vi "KioskDemoHoriz.vi"() -> ()   [LabVIEW 2023]
doc: "DESCRIPTION\nGeneral Application \n\nVERSION\nD1:00\nFirst Release To customer\nDD/MM/YYYY\n\nTemplate D2:01\nMade lighter and simpler\n14-04-2020"
uses:
  SubVIs/Controls/SetupModeState.ctl
  <vilib>/event_ctls.llb/eventsource.ctl
  <vilib>/Utility/miscctls.llb/LVBoundsTypeDef.ctl
  SubVIs/Controls/DisplayQCommand.ctl
  SubVIs/Controls/QueueCommand.ctl
  SubVIs/Controls/DisplayMessage.ctl
  SubVIs/Controls/Transition.ctl
  SubVIs/utilities/Error/ErrorCommand.ctl
  SubVIs/Controls/Tab.ctl
  SubVIs/Controls/StateMessage.ctl
  SubVIs/Error/ErrorMessage.ctl
  SubVIs/utilities/Config/System Config Data Manager Parameter.ctl
  SubVIs/utilities/Config/ConfigCommand.ctl
  SubVIs/Buttons/ButtonCommands.ctl
  SubVIs/Buttons/MenuType.ctl
panel:
  in  "Position:Top":i32
  in  "exit":bool
  in  "Container Bounds":T1
  out "Application Directory":path
  in  "ButtonsMenu":enum32{"Page 1"}(tab)
  out "SubmenuVisible":bool
  out "State":T2=enum."Initialising"
  out "UI Output":string
  out "Menu Output":string
  in  "Tab Control 2":enum32{"Page 1", "Page 4", "Page 2", "Page 3"}(tab)
  in  "Stop":bool
  in  "Source":T3 items=["LabVIEW UI"=0, "ActiveX"=1, "User Event"=25]
  in  "Start":bool
  out "ErrorHandlingLoop":i32
  out "StateMachineLoop":i32
  out "UILoop":i32
  out "EventLoop":i32
  in  "Main Screen Tabs":enum32{"Main Screen"}(tab)
  out "Tab Control":T4(tab)
  in  "Error Loop":enum16{"Event Loop", "UI Q Loop", "State Loop"}(ring)
  in  "Generate Error":bool
  out "EngMode?":bool
  in  "Enter Password":string
  out "ConfigdB path":path
  in  "Home Button":bool
  in  "ErrorLog":bool
  in  "Clear Alarm":bool
  in  "ErrorLog":i32(listbox)
  out "Error":string
  out "ErrorIndicator":bool
  in  "ViewError":bool
  out "Version":string
  out "Time":string
  out "Status":string
  # "GenAppMain"
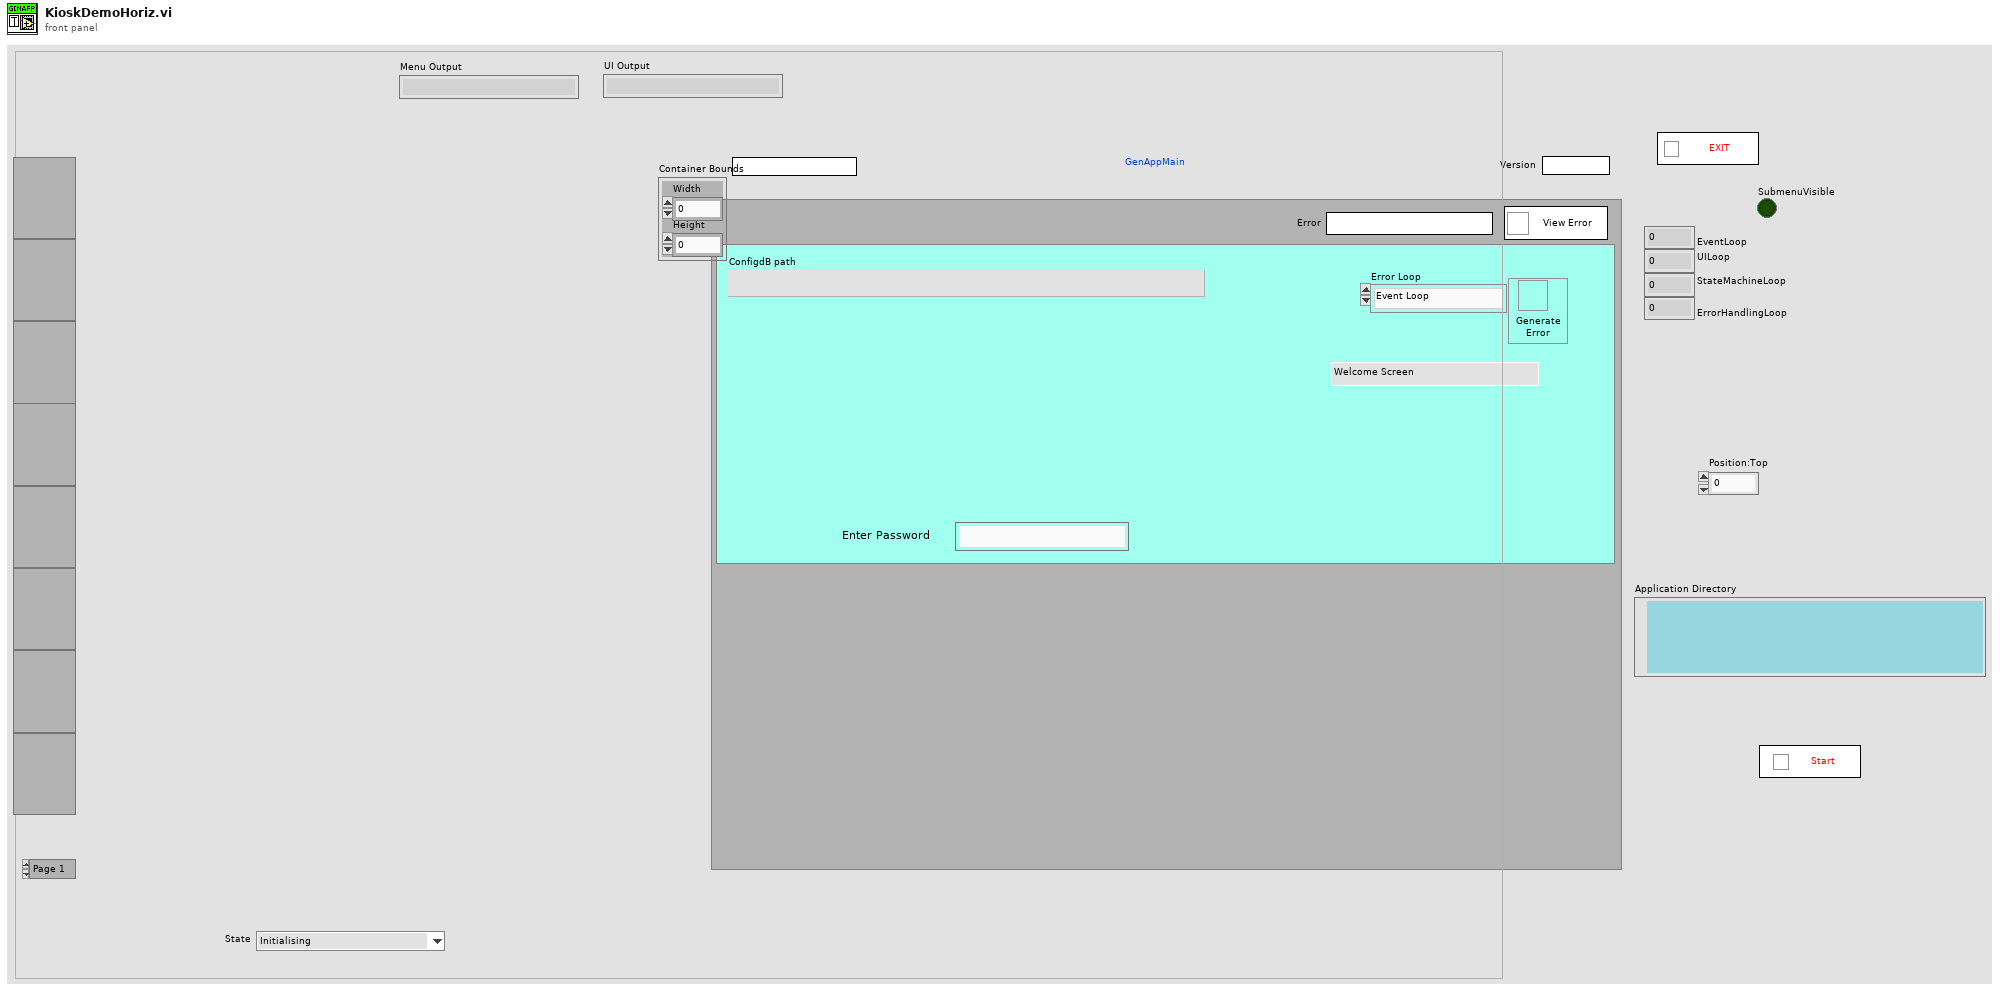
[diagram p1: front panel]
types:
  T1 = typedef "LVBoundsTypeDef.ctl" = cluster{"Width":u32, "Height":u32}
  T2 = typedef "SetupModeState.ctl" = enum16{"No State - Error", "Initialising", "Idling", "Running", "Sorting Menu", "Resetting Menu", "Sorting Submenu", "Loading UI", "Erroring", "Exiting"}
  T3 = typedef "eventsource.ctl" = u32
  T4 = enum32{"Welcome Screen", "Eng Set Up", "Oppo Run Screen", "Eng Run Screen", "Test Report Screen", "Error"}
  T5 = typedef "DisplayQCommand.ctl" = enum16{"No Command - Error", "Initialise", "Get Q Reference", "Add Item to Bottom", "Add Item to Top", "Flush Q", "Dequeue", "Peek Next Element", "Close"}
  T6 = typedef "QueueCommand.ctl" = enum16{"No Command - Error", "Initialise", "Add to Bottom", "Add To Top", "Get Ref", "Close"}
  T7 = typedef "ErrorCommand.ctl" = enum16{"No Command - Error", "Set to Dev Mode", "Set To Released Mode", "Set Error", "Log Error", "Throw Error", "Log & Throw Error", "Set Error Timed"}
  T8 = enum32{"invalid app kind", "Development System", "Run Time System", "Student Edition", "Embedded LabVIEW", "Evaluation", "Custom"}
  T9 = typedef "DisplayMessage.ctl" = enum16{"No Message - Ignore", "Display Message", "Set Tab", "Set Status", "Add Error Message", "Clear Error History", "Generate Error", "Set Idling Display", "Set Running Display", "Set Subpanel Output", "Stop"}
  T10 = typedef "ErrorMessage.ctl" = enum16{"No Message - Ignore", "Display Message", "Stop"}
  T11 = typedef "StateMessage.ctl" = cluster{"Transition":T12, "variant":variant}
  T12 = typedef "Transition.ctl" = enum16{"No Transition - Error", "Initialise", "Login", "Authenticate", "Log on Fail", "Login Success", "Logout", "Generate Error", "Start", "Stop", "Menu Button Pressed", "UI Button Pressed", "Exit"}
  T13 = typedef "ConfigCommand.ctl" = enum16{"No Command - Error", "Initialise Config SQLite", "Save Config", "Get Key", "Set Key", "Update Key", "Get Latest Config Data", "Get Config Data for Version", "Get Default Config Data"}
  T14 = typedef "System Config Data Manager Parameter.ctl" = enum16{"Eng Password", "DSN Connection", "User Password", "RunStatus", "InitialDataPath", "helpFilePath", "ErrorFilepath", "DatalogPath", "Hello"}
  T15 = typedef "Tab.ctl" = enum32{"Welcome Screen", "Eng Set Up", "Oppo Run Screen", "Eng Run Screen", "Test Report Screen", "Error"}
  T16 = typedef "lveventtype.ctl" = enum32{"Null", "Timeout", "Annotation Menu Selection", "Annotation Menu Selection?", "App Instance Close", "App Instance Close?", "Autoscale Range Change", "Bookmark Info Change", "Cell Edit", "Cell Edit?", "Cursor Grab", "Cursor Grab?", "Cursor Menu Selection", "Cursor Menu Selection?", "Cursor Move", "Cursor Release", "Data Change", "Direction Change", "Display State Change", "Drag Ended", "Drag Enter", "Drag Leave", "Drag Over", "Drag Source Update", "Drag Starting", "Drag Starting?", "Drop", "Exec State Change", "Key Down", "Key Down?", "Key Repeat", "Key Repeat?", "Key Up", "Listbox Double Click", "Menu Activation?", "Menu Selection (App)", "Menu Selection? (App)", "Menu Selection (User)", "Mouse Down", "Mouse Down?", "Mouse Enter", "Mouse Leave", "Mouse Move", "Mouse Up", "Mouse Wheel", "NI Security User Change (App)", "Pane Size", "Panel Close", "Panel Close?", "Panel Resize", "Plot Attribute Change", "Scale Range Change", "Shortcut Menu Activation?", "Shortcut Menu Selection (App)", "Shortcut Menu Selection? (App)", "Shortcut Menu Selection (User)", "Tree Double Click", "Tree Drag", "Tree Drag?", "Tree Drop", "Tree Drop?", "Tree Item Close", "Tree Item Close?", "Tree Item Open", "Tree Item Open?", "User Event", "Value Change"}
  T17 = typedef "MenuType.ctl" = enum16{"Main", "Simulation", "ME", "SF", "User Utilities", "Dev Tools"}
  T18 = typedef "ButtonCommands.ctl" = enum16{"No Command - Error", "Load Buttons", "Remove Buttons"}
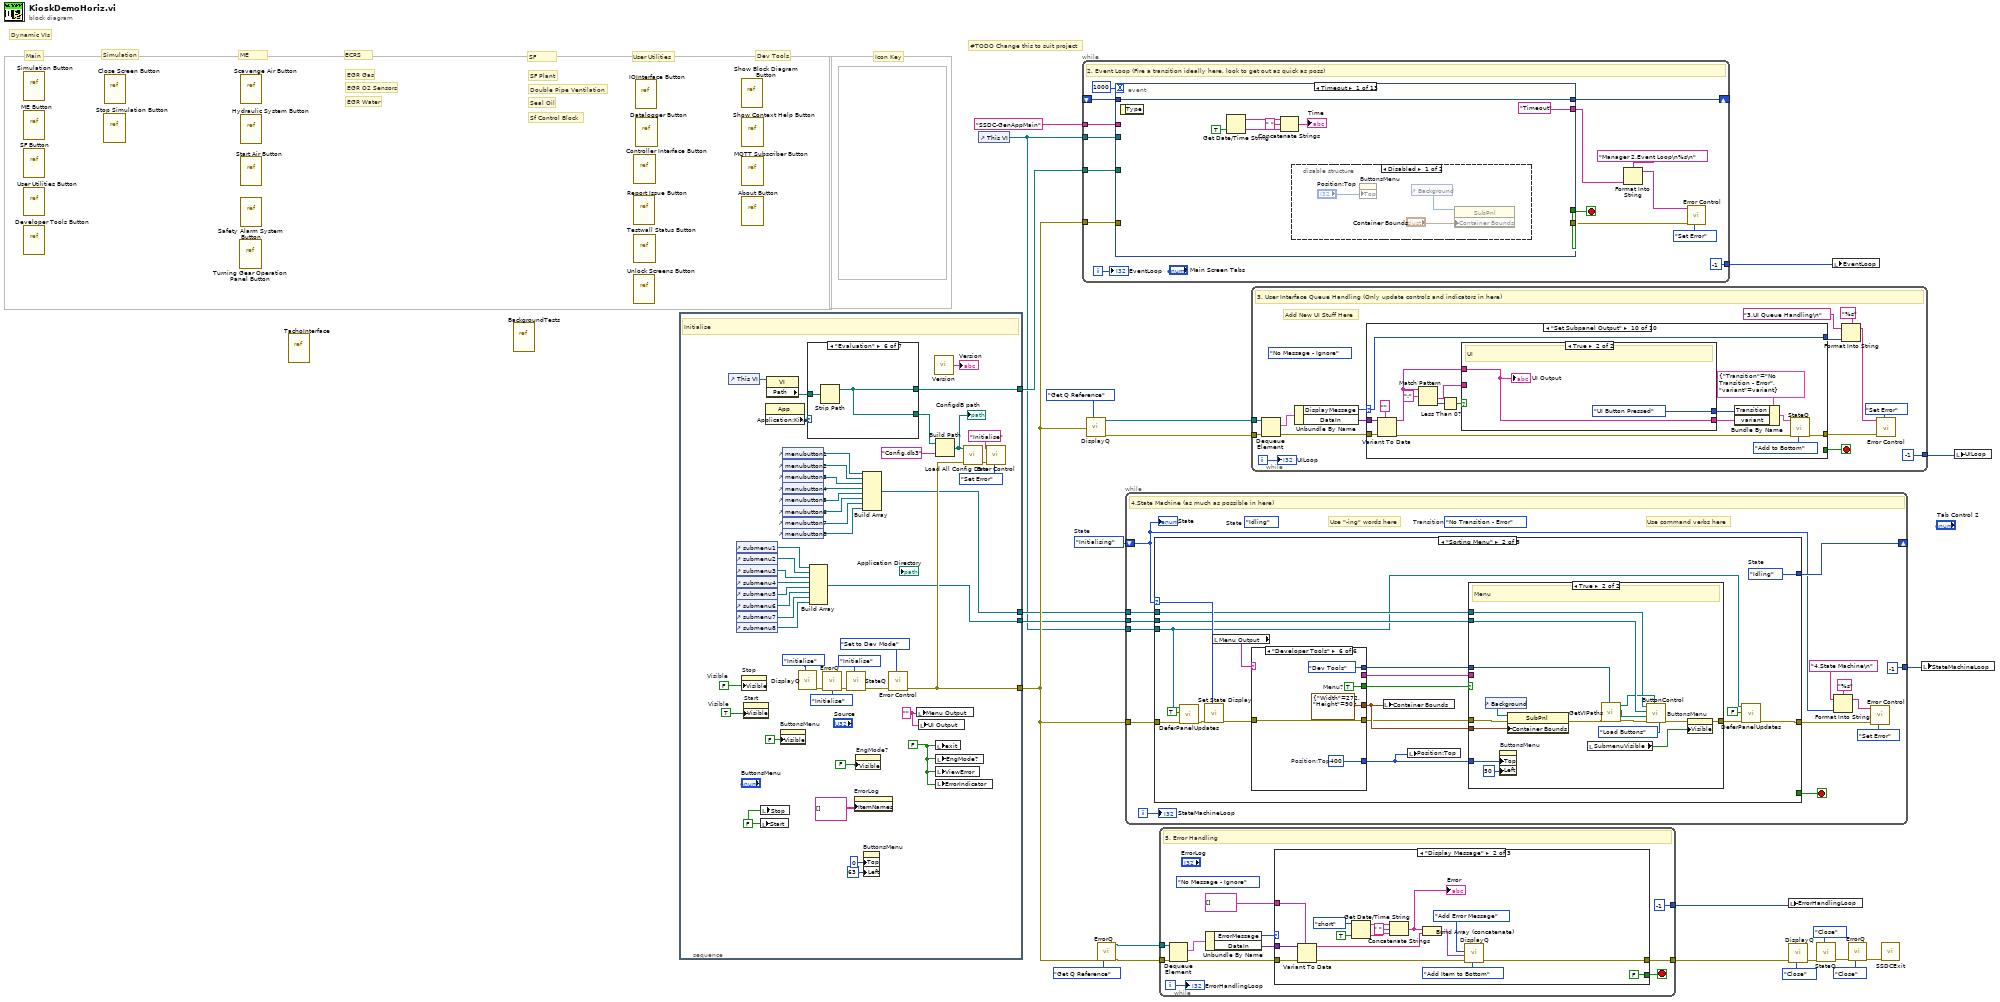
[diagram p0: block diagram]
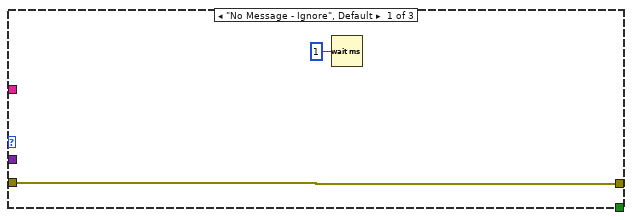
[diagram p2: hidden frame]
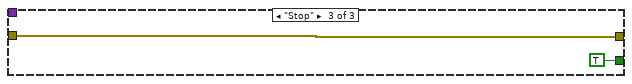
[diagram p3: hidden frame]
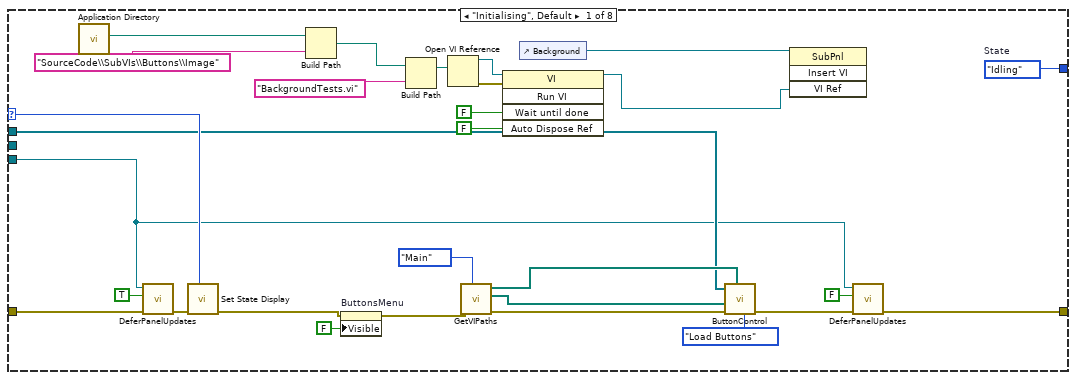
[diagram p4: hidden frame]
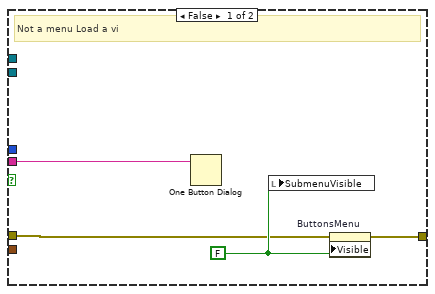
[diagram p5: hidden frame]
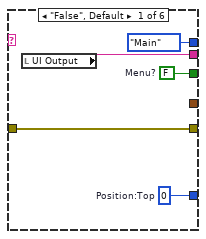
[diagram p6: hidden frame]
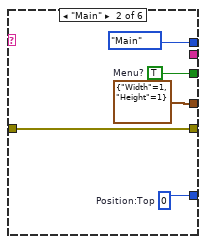
[diagram p7: hidden frame]
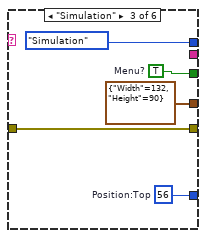
[diagram p8: hidden frame]
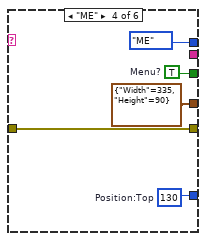
[diagram p9: hidden frame]
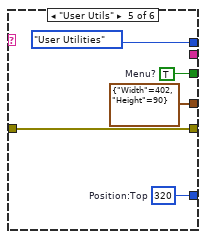
[diagram p10: hidden frame]
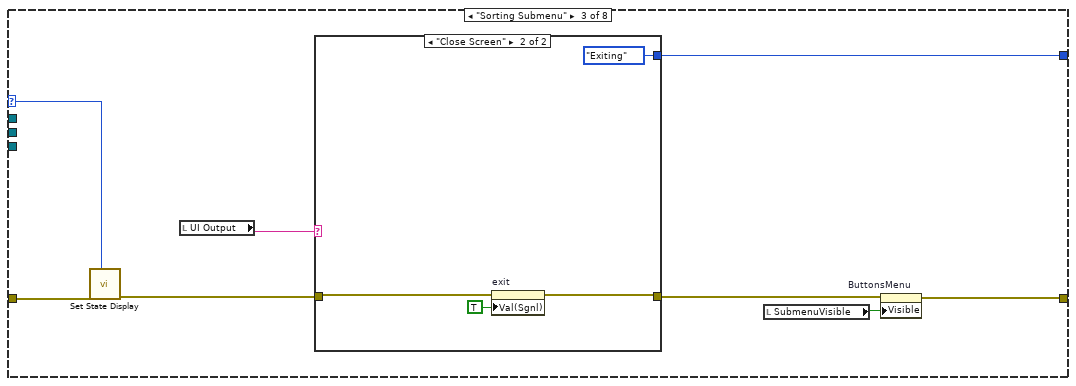
[diagram p11: hidden frame]
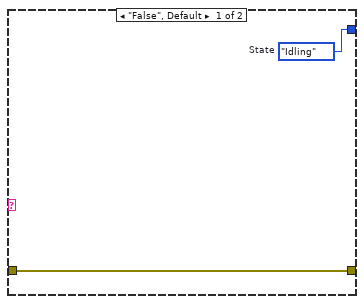
[diagram p12: hidden frame]
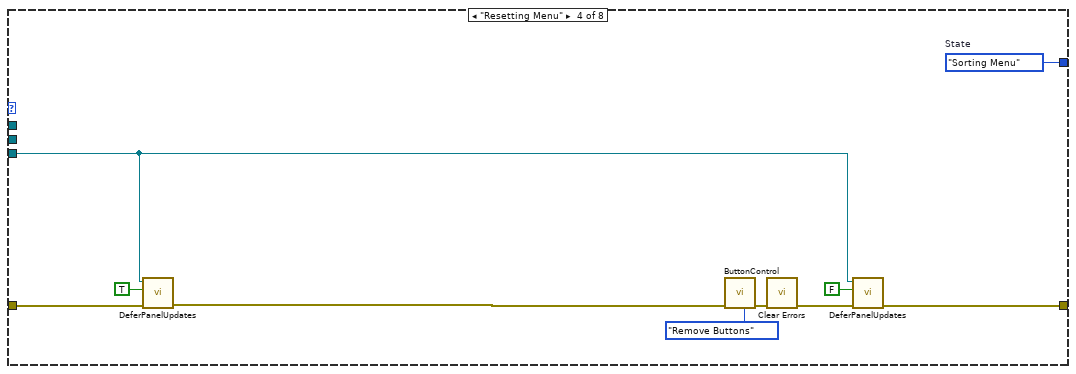
[diagram p13: hidden frame]
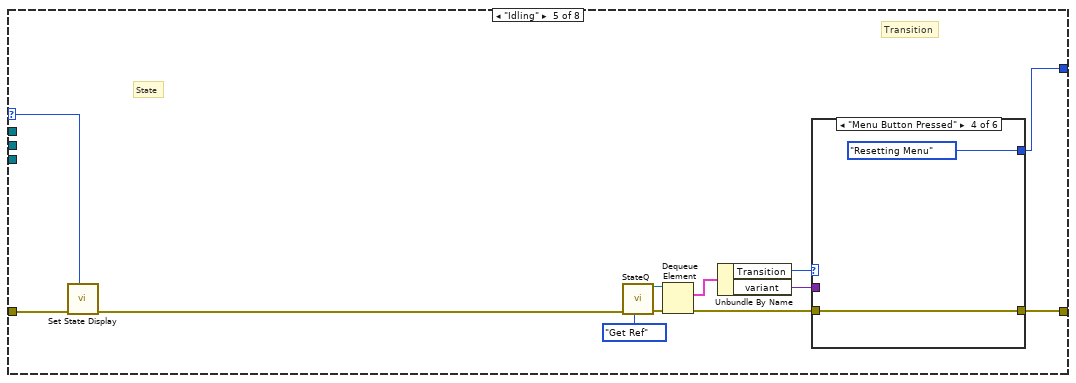
[diagram p14: hidden frame]
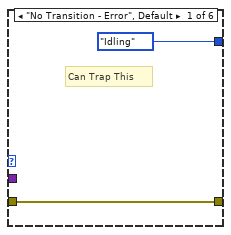
[diagram p15: hidden frame]
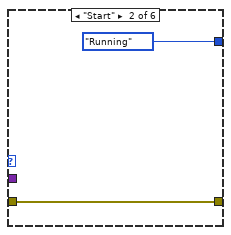
[diagram p16: hidden frame]
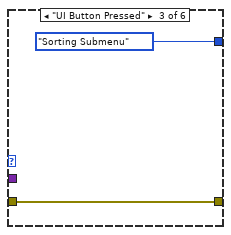
[diagram p17: hidden frame]
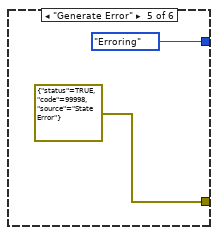
[diagram p18: hidden frame]
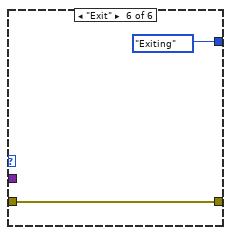
[diagram p19: hidden frame]
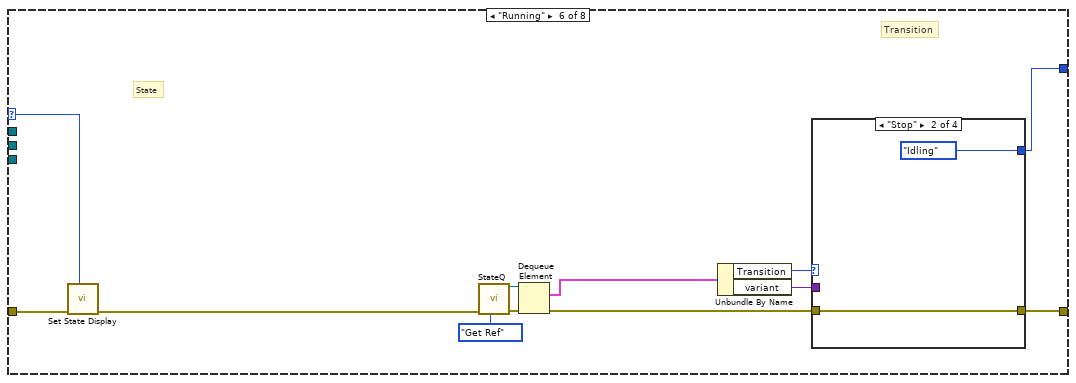
[diagram p20: hidden frame]
diagram:
  w24 = SetupModeState."Initialising"  # State
  # "Sf Control Block"
  # "Seal Oil"
  # "Double Pipe Ventilation"
  # "SF Plant"
  # "SF"
  # "EGR Water"
  # "EGR O2 Sensors"
  # "EGR Gas"
  # "ECRS"
  # "Dev Tools"
  # "User Utilities"
  # "Main"
  # "Simulation"
  # "ME"
  # "Dynamic VIs"
  # "#TODO Change this to suit project"
  # "Icon Key"
  n1 = vi-ref "Simulation Button.vi"() -> ()  [unwired: 1 out]
  n2 = vi-ref "ME Button.vi"() -> ()  [unwired: 1 out]
  n3 = vi-ref "SF Button.vi"() -> ()  [unwired: 1 out]
  n4 = vi-ref "User Utilities Button.vi"() -> ()  [unwired: 1 out]
  n5 = vi-ref "Developer Tools Button.vi"() -> ()  [unwired: 1 out]
  n6 = vi-ref "Stop Simulation Button.vi"() -> ()  [unwired: 1 out]
  n7 = vi-ref "Close Screen Button.vi"() -> ()  [unwired: 1 out]
  n8 = vi-ref "Turning Gear Operation Panel Button.vi"() -> ()  [unwired: 1 out]
  n9 = vi-ref "Scavenge Air Button.vi"() -> ()  [unwired: 1 out]
  n10 = vi-ref "Hydraulic System Button.vi"() -> ()  [unwired: 1 out]
  n11 = vi-ref "Start Air Button.vi"() -> ()  [unwired: 1 out]
  n12 = vi-ref "Safety Alarm System Button.vi"() -> ()  [unwired: 1 out]
  n13 = vi-ref "TachoInterface.vi"() -> ()  [unwired: 1 out]
  n14 = vi-ref "BackgroundTests.vi"() -> ()  [unwired: 1 out]
  n15 = vi-ref "Report Issue Button.vi"() -> ()  [unwired: 1 out]
  n16 = vi-ref "Unlock Screens Button.vi"() -> ()  [unwired: 1 out]
  n17 = vi-ref "Controller Interface Button.vi"() -> ()  [unwired: 1 out]
  n18 = vi-ref "Testwall Status Button.vi"() -> ()  [unwired: 1 out]
  n19 = vi-ref "IOInterface Button.vi"() -> ()  [unwired: 1 out]
  n20 = vi-ref "Datalogger Button.vi"() -> ()  [unwired: 1 out]
  n21 = stacked-sequence "1. Initialisation" {
    tunnel: [w50] -> w11
    tunnel: [w55] -> w19
    tunnel: [w39] -> w3
    tunnel: [w31] -> w2
    frame #0 {
      w29 = "" ("Menu Output")
      w48 = FALSE  # Visible
      w47 = TRUE  # Visible
      w53 = FALSE ("Stopped")
      w49 = FALSE ("Start")
      # "Initialise"
      n22 = control-ref of="This VI"() -> (w66:refnum<vi>)
      n23 = control-ref of="submenu1"() -> (w38:refnum<vi>)
      n24 = control-ref of="submenu2"() -> (w37:refnum<vi>)
      n25 = control-ref of="submenu3"() -> (w36:refnum<vi>)
      n26 = control-ref of="submenu4"() -> (w35:refnum<vi>)
      n27 = control-ref of="submenu5"() -> (w34:refnum<vi>)
      n28 = control-ref of="submenu6"() -> (w33:refnum<vi>)
      n29 = control-ref of="submenu7"() -> (w32:refnum<vi>)
      n30 = control-ref of="submenu8"() -> (w28:refnum<vi>)
      n31 = property on="Stop" class="Bool (strict)"("Visible"=w48) -> ()  [unwired: 2 in, 2 out]
      n32 = property on="Start" class="Bool (strict)"("Visible"=w47) -> ()  [unwired: 2 in, 2 out]
      n33 = local write "Start"(w49) -> ()
      n34 = local write "Stop"(w49) -> ()
      n35 = property class="App"() -> ("Application:Kind"=w65:T8)  [unwired: 2 in, 2 out]
      n36 = property class="VI"(reference=w66) -> ("Path"=w67:path)  [unwired: 1 in, 2 out]
      n37 = property on="ButtonsMenu" class="TabCtl (strict)"("Visible"=FALSE) -> ()  [unwired: 2 in, 2 out]
      n38 = control-ref of="menubutton1"() -> (w41:refnum<vi>)
      n39 = control-ref of="menubutton2"() -> (w40:refnum<vi>)
      n40 = control-ref of="menubutton3"() -> (w46:refnum<vi>)
      n41 = control-ref of="menubutton4"() -> (w45:refnum<vi>)
      n42 = control-ref of="menubutton5"() -> (w44:refnum<vi>)
      n43 = control-ref of="menubutton6"() -> (w43:refnum<vi>)
      n44 = control-ref of="menubutton7"() -> (w42:refnum<vi>)
      n45 = control-ref of="menubutton8"() -> (w30:refnum<vi>)
      n46 = call "DisplayQ.vi"("command"=DisplayQCommand."Initialise") -> ("error out"=w60:errorcluster)  [unwired: 4 in, 3 out]
      n47 = case shown="\"Evaluation\"" w65 {
        tunnel: w67 -> [w72 w74 w78 w81 w83 w85 w87]
        tunnel: [w72 w73 w77 w80 w82 w84 w86] -> w56
        tunnel: [w72 w73 w75 w80 w82 w84 w86] -> w55
        frame "invalid app kind", Default {
        }
        frame "Development System" {
          n48 = Strip Path(path=w74) -> (stripped path=w73:path)  [unwired: 1 out]
        }
        frame "Run Time System" {
          n49 = Strip Path(path=w78) -> (stripped path=w79:path)  [unwired: 1 out]
          n50 = Strip Path(path=w79) -> (stripped path=w75:path)  [unwired: 1 out]
          n51 = Build Path(base path=w75, name or relative path="data") -> (appended path=w77:path)
        }
        frame "Student Edition" {
          n52 = Strip Path(path=w81) -> (stripped path=w80:path)  [unwired: 1 out]
        }
        frame "Embedded LabVIEW" {
          n53 = Strip Path(path=w83) -> (stripped path=w82:path)  [unwired: 1 out]
        }
        frame "Evaluation" {
          n54 = Strip Path(path=w85) -> (stripped path=w84:path)  [unwired: 1 out]
        }
        frame "Custom" {
          n55 = Strip Path(path=w87) -> (stripped path=w86:path)  [unwired: 1 out]
        }
      }
      n56 = Build Array(w38, w37, w36, w35, w34, w33, w32, w28) -> (w31:refnum<vi>[])
      n57 = call "ErrorQ.vi"("command"=DisplayQCommand."Initialise", "error in (no error)"=w60) -> ("error out"=w61:errorcluster)  [unwired: 3 in, 3 out]
      n58 = call "StateQ.vi"("QueueCommand"=QueueCommand."Initialise", "error in (no error)"=w61) -> ("error out"=w51:errorcluster)  [unwired: 5 in, 1 out]
      n59 = property on="ErrorLog" class="MCListbox (strict)"("ItemNames"=string[][] [] ("Item Names")) -> ()  [unwired: 2 in, 2 out]
      n60 = property on="EngMode?" class="Bool (strict)"("Visible"=FALSE) -> ()  [unwired: 2 in, 2 out]
      n61 = Build Array(w41, w40, w46, w45, w44, w43, w42, w30) -> (w39:refnum<vi>[])
      n62 = property on="ButtonsMenu" class="TabCtl (strict)"("Top"=0 ("Position:Top"), "Left"=63 ("Position:Left")) -> ()  [unwired: 2 in, 2 out]
      n63 = call "Error Control.vi"("Command"=ErrorCommand."Set to Dev Mode", "error in (no error)"=w51) -> ("error out"=w50:errorcluster)  [unwired: 6 in]
      n64 = local write "Menu Output"(w29) -> ()
      n65 = local write "UI Output"(w29) -> ()
      n66 = call "Version.vi"() -> ("Version"=→"Version":string)  [unwired: 5 in]
      n67 = local write "exit"(w53) -> ()
      n68 = local write "ViewError"(w53) -> ()
      n69 = local write "ErrorIndicator"(w53) -> ()
      n70 = Build Path(base path=w56, name or relative path="Config.db3") -> (appended path=w68:path)
      "ConfigdB path" <- w68
      n71 = local write "EngMode?"(w53) -> ()
      n72 = call "Load All Config Data.vi"("error in (no error)"=w50, "path"=w68) -> ("error out"=w58:errorcluster)  [unwired: 5 in]
      n73 = call "Error Control.vi"("Command"=ErrorCommand."Set Error", "error in (no error)"=w58, "Source"="Initialise") -> ()  [unwired: 5 in, 1 out]
    }
  }
  n74 = vi-ref "Show Block Diagram Button.vi"() -> ()  [unwired: 1 out]
  n75 = vi-ref "Show Context Help Button.vi"() -> ()  [unwired: 1 out]
  n76 = vi-ref "MQTT Subscriber Button.vi"() -> ()  [unwired: 1 out]
  n77 = vi-ref "About Button.vi"() -> ()  [unwired: 1 out]
  n78 = control-ref of="This VI"() -> (w1:refnum<vi>)
  n79 = while "2. Event Loop" {
    tunnel: w11 -> [w99]
    shift-right: [w96] -> _
    shift-left: _ -> [w95]
    tunnel: w1 -> [w94]
    tunnel: [-1 ("ErrorHandlingLoop")] -> w20
    tunnel: w19 -> [w92]
    tunnel: "SSDC-GenAppMain" ("name or relative path") -> [w91]
    i -> [w102]
    stop <- w101 stop-if-true
    # "2. Event Loop (Fire a transition ideally here, look to get out as quick as poss)"
    n80 = event shown="[0] Timeout" {
      selector: _ -> [_ _ _ _ _ _ _ _ _ _ _ _ _]
      dyn-events: _ -> [_ _ _ _ _ _ _ _ _ _ _ _ _]
      timeout: 1000 -> [_ _ _ _ _ _ _ _ _ _ _ _ _]
      tunnel: [_ FALSE ("STOP?") _ TRUE ("STOP?") _ _ _ w189 _ _ _ _ _] -> w101
      tunnel: w99 -> [_ w115 _ _ w147 w162 _ w186 w206 w224 w237 w260 _]
      tunnel: [_ w115 _ _ w146 w161 _ w185 w205 w223 w236 w259 _] -> w97
      tunnel: ["Timeout" "Panel Close?" ("Event") w119 w126 w143 w157 w171 w180 w198 w217 w230 w253 w272] -> w88
      tunnel: [w105 w114 w124 w129 w150 w164 w174 w188 w201 w222 w233 w261 w276] -> w96
      tunnel: w95 -> [w105 w114 w124 w129 w150 w164 w174 w188 _ w222 w233 w261 w276]
      tunnel: w94 -> [_ _ _ _ _ _ _ w187 _ _ _ _ w275]
      tunnel: w92 -> [_ _ _ _ _ _ _ w184 _ _ _ _ _]
      tunnel: w91 -> [_ _ _ _ _ _ _ _ _ _ _ _ _]
      event Timeout {
        n81 = event-data() -> ()  [unwired: 1 in, 1 out]
        n82 = Get Date/Time String(want seconds? (F)=TRUE) -> (date string=w108:string, time string=w107:string)  [unwired: 2 in]
        n83 = Concatenate Strings(w108, " " ("string"), w107) -> (→"Time":string)
        n84 = disable-structure shown="Disabled" {
          frame Disabled {
            n85 = property on="ButtonsMenu" class="TabCtl (strict)"("Top"="Position:Top") -> ()  [unwired: 2 in, 2 out]
            n86 = control-ref of="Background"() -> (w111:refnum<vi>)
            n87 = property class="SubPnl"(reference=w111, "Container Bounds"="Container Bounds") -> ()  [unwired: 1 in, 2 out]
          }
          frame Enabled {
          }
        }
      }
      event Panel Close? {
        n88 = event-data() -> ()  [unwired: 1 in, 1 out]
        n89 = property on="exit" class="Bool (strict)"("Val(Sgnl)"=TRUE ("Value (Signaling)")) -> ()  [unwired: 2 in, 2 out]
        n90 = event-data("Discard?"=TRUE) -> ()  [unwired: 1 in, 1 out]
      }
      event "ErrorLog": Value Change {
        n91 = event-data() -> ("CtlRef"=w121:refnum<vi>, "Type"=w120:T16)  [unwired: 1 in]
        n92 = call "CreateEventString.vi"("Type in"=w120, "Ctl Refnum"=w121) -> ("Event"=w119:string)  [unwired: 9 in]
        n93 = case shown="True" "ErrorLog" {
          tunnel: [_ FALSE] -> w122
          frame False {
          }
          frame True {
            n94 = call "ErrorLogDialog.vi"() -> ()  [unwired: 11 in, 1 out]
          }
        }
        n95 = local write "ErrorLog"(w122) -> ()
      }
      event "exit": Value Change {
        n96 = event-data() -> ("CtlRef"=w128:refnum<vi>, "Type"=w127:T16)  [unwired: 1 in]
        n97 = local write "Start"(FALSE ("Start")) -> ()
        n98 = call "CreateEventString.vi"("Type in"=w127, "Ctl Refnum"=w128) -> ("Event"=w126:string)  [unwired: 9 in]
        n99 = stacked-sequence {
          tunnel: [_ FALSE] -> w130
          frame #0 {
            n100 = call "StateQ.vi"("QueueCommand"=QueueCommand."Add To Top", "output cluster"=T11 {"Transition"=enum."Exit", "variant"=variant}) -> ("error out"=w137:errorcluster)  [unwired: 5 in, 1 out]
            n101 = call "ErrorQ.vi"("command"=DisplayQCommand."Add Item to Top", "error in (no error)"=w137, "ErrorMessage"=ErrorMessage."Stop") -> ("error out"=w134:errorcluster)  [unwired: 2 in, 3 out]
            n102 = call "DisplayQ.vi"("command"=DisplayQCommand."Add Item to Top", "error in (no error)"=w134, "DisplayMessage"=DisplayMessage."Stop") -> ()  [unwired: 2 in, 4 out]
          }
          frame #1 {
            n103 = Wait (ms)(milliseconds to wait=u32 500) -> ()  [unwired: 1 out]
          }
        }
        n104 = local write "exit"(w130) -> ()
      }
      event "Start": Value Change {
        n105 = event-data() -> ("CtlRef"=w145:refnum<vi>, "Type"=w144:T16)  [unwired: 1 in]
        n106 = call "CreateEventString.vi"("Type in"=w144, "Ctl Refnum"=w145) -> ("Event"=w143:string)  [unwired: 9 in]
        n107 = case shown="True" "Start" {
          tunnel: [_ FALSE ("Start")] -> w148
          tunnel: w147 -> [w151 w153]
          tunnel: [w151 w152] -> w146
          frame False {
          }
          frame True {
            n108 = call "StateQ.vi"("QueueCommand"=QueueCommand."Add To Top", "error in (no error)"=w153, "output cluster"=T11 {"Transition"=enum."Start", "variant"=variant}) -> ("error out"=w152:errorcluster)  [unwired: 4 in, 1 out]
          }
        }
        n109 = local write "Start"(w148) -> ()
      }
      event "Stop": Value Change {
        n110 = event-data() -> ("CtlRef"=w159:refnum<vi>, "Type"=w158:T16)  [unwired: 1 in]
        n111 = call "CreateEventString.vi"("Type in"=w158, "Ctl Refnum"=w159) -> ("Event"=w157:string)  [unwired: 9 in]
        n112 = case shown="True" "Stop" {
          tunnel: [_ FALSE ("Start")] -> w163
          tunnel: w162 -> [w165 w167]
          tunnel: [w165 w166] -> w161
          frame False {
          }
          frame True {
            n113 = call "StateQ.vi"("QueueCommand"=QueueCommand."Add To Top", "error in (no error)"=w167, "output cluster"=T11 {"Transition"=enum."Stop", "variant"=variant}) -> ("error out"=w166:errorcluster)  [unwired: 4 in, 1 out]
          }
        }
        n114 = local write "Stop"(w163) -> ()
      }
      event "Enter Password": Value Change {
        n115 = event-data() -> ("CtlRef"=w173:refnum<vi>, "Type"=w172:T16)  [unwired: 1 in]
        n116 = call "CreateEventString.vi"("Type in"=w172, "Ctl Refnum"=w173) -> ("Event"=w171:string)  [unwired: 9 in]
        n117 = call "SQLiteConfig.vi"("ConfigCommand"=ConfigCommand."Get Key", "Parameter"=System_Config_Data_Manager_Parameter."Eng Password") -> ("KeyData"=w175:string)  [unwired: 3 in, 3 out]
        n118 = Equal?(x=w175, y="Enter Password") -> (x = y?=w179:bool)
        "EngMode?" <- w179
        n119 = property on="EngMode?" class="Bool (strict)"("Visible"=w179) -> ()  [unwired: 2 in, 2 out]
      }
      event Menu Selection (User) {
        n120 = event-data() -> ("Type"=w182:T16, "ItemTag"=w181:string)  [unwired: 1 in]
        n121 = Format Into String(format string="\"Menu\":%s:%s", w182, w181) -> (resulting string=w180:string)  [unwired: 2 in, 1 out]
        n122 = case shown="\"About\"" w181 {
          tunnel: [_ FALSE _ _] -> w189
          tunnel: w187 -> [_ _ _ w197]
          tunnel: w186 -> [w190 w191 w194 w195]
          tunnel: [w190 w191 w194 w195] -> w185
          tunnel: w184 -> [_ _ _ _]
          frame "False", Default {
          }
          frame "Exit" {
            n123 = property on="exit" class="Bool (strict)"("Val(Sgnl)"=TRUE ("Value (Signaling)")) -> ()  [unwired: 2 in, 2 out]
          }
          frame "Configuration" {
            n124 = call "ConfigSQLiteSettingDialog.vi"() -> ()  [unwired: 1 in]
          }
          frame "About" {
            n125 = property class="VI"(reference=w197) -> ("Description"=w196:string)  [unwired: 1 in, 2 out]
            n126 = call "AboutScreen.vi"("Version Info. In"=w196) -> ()  [unwired: 11 in]
          }
        }
      }
      event "ViewError": Value Change {
        n127 = event-data() -> ("CtlRef"=w199:refnum<vi>, "Type"=w200:T16)  [unwired: 1 in]
        n128 = local read "Tab Control"() -> (w202:T4)
        n129 = call "CreateEventString.vi"("Type in"=w200, "Ctl Refnum"=w199) -> ("Event"=w198:string)  [unwired: 9 in]
        n130 = case shown="True" "ViewError" {
          tunnel: w206 -> [w209 w213]
          tunnel: [w209 w212] -> w205
          tunnel: [FALSE FALSE] -> w203
          tunnel: w202 -> [w207 w210]
          tunnel: [w207 w210] -> w201
          frame False {
          }
          frame True {
            n131 = call "DisplayQ.vi"("command"=DisplayQCommand."Add Item to Bottom", "error in (no error)"=w213, "DataIn"=Tab."Error" ("Tab Control"), "DisplayMessage"=DisplayMessage."Set Tab") -> ("error out"=w212:errorcluster)  [unwired: 1 in, 3 out]
          }
        }
        n132 = local write "ViewError"(w203) -> ()
      }
      event "Clear Alarm": Value Change {
        n133 = event-data() -> ("CtlRef"=w218:refnum<vi>, "Type"=w219:T16)  [unwired: 1 in]
        n134 = call "CreateEventString.vi"("Type in"=w219, "Ctl Refnum"=w218) -> ("Event"=w217:string)  [unwired: 9 in]
        n135 = case shown="True" "Clear Alarm" {
          tunnel: w224 -> [w226 w228]
          tunnel: [w226 w228] -> w223
          tunnel: [FALSE FALSE] -> w220
          frame False {
          }
          frame True {
            n136 = local write "ErrorIndicator"(FALSE ("ErrorIndicator")) -> ()
          }
        }
        n137 = local write "Clear Alarm"(w220) -> ()
      }
      event "Home Button": Value Change {
        n138 = event-data() -> ("CtlRef"=w232:refnum<vi>, "Type"=w231:T16)  [unwired: 1 in]
        n139 = call "CreateEventString.vi"("Type in"=w231, "Ctl Refnum"=w232) -> ("Event"=w230:string)  [unwired: 9 in]
        n140 = case shown="True" "Home Button" {
          tunnel: w237 -> [w239 w244]
          tunnel: [w239 w243] -> w236
          tunnel: [FALSE FALSE] -> w235
          tunnel: w233 -> [_ w241]
          frame False {
          }
          frame True {
            n141 = case shown="\"Error\"" w241 {
              tunnel: [Tab."Welcome Screen" ("Tab Control") Tab."Oppo Run Screen" ("Tab Control") Tab."Eng Run Screen" ("Tab Control") Tab."Test Report Screen" ("Tab Control") Tab."Error" ("Tab Control") Tab."Eng Run Screen" ("Tab Control")] -> w240
              frame "Welcome Screen" {
              }
              frame "Oppo Run Screen" {
              }
              frame "Eng Run Screen" {
              }
              frame "Test Report Screen" {
              }
              frame "Error" {
              }
              frame "Eng Set Up" {
              }
            }
            n142 = call "DisplayQ.vi"("command"=DisplayQCommand."Add Item to Bottom", "error in (no error)"=w244, "DataIn"=w240, "DisplayMessage"=DisplayMessage."Set Tab") -> ("error out"=w243:errorcluster)  [unwired: 1 in, 3 out]
          }
        }
        n143 = local write "Home Button"(w235) -> ()
      }
      event "Generate Error": Value Change {
        n144 = event-data() -> ("CtlRef"=w255:refnum<vi>, "Type"=w254:T16)  [unwired: 1 in]
        n145 = call "CreateEventString.vi"("Type in"=w254, "Ctl Refnum"=w255) -> ("Event"=w253:string)  [unwired: 9 in]
        n146 = case shown="\"UI Q Loop\"" "Error Loop" {
          tunnel: w260 -> [_ w264 w269]
          tunnel: [errorcluster {"status"=TRUE, "code"=99999, "source"="Random Event Error"} ("error out") w263 w270] -> w259
          tunnel: "Generate Error" -> [_ _ _]
          tunnel: [_ _ FALSE] -> w256
          frame "Event Loop", Default {
          }
          frame "UI Q Loop" {
            n147 = call "DisplayQ.vi"("command"=DisplayQCommand."Add Item to Bottom", "error in (no error)"=w264, "DisplayMessage"=DisplayMessage."Generate Error") -> ("error out"=w263:errorcluster)  [unwired: 2 in, 3 out]
          }
          frame "State Loop" {
            n148 = call "StateQ.vi"("QueueCommand"=QueueCommand."Add to Bottom", "error in (no error)"=w269, "output cluster"=T11 {"Transition"=enum."Generate Error", "variant"=variant}) -> ("error out"=w270:errorcluster)  [unwired: 4 in, 1 out]
          }
        }
        n149 = local write "Generate Error"(w256) -> ()
      }
      event "Version": Mouse Down {
        n150 = event-data() -> ("CtlRef"=w274:refnum<vi>, "Type"=w273:T16)  [unwired: 1 in]
        n151 = call "CreateEventString.vi"("Type in"=w273, "Ctl Refnum"=w274) -> ("Event"=w272:string)  [unwired: 9 in]
        n152 = property class="VI"(reference=w275) -> ("Description"=w277:string)  [unwired: 1 in, 2 out]
        n153 = call "VIDescription.vi"("VersionData In"=w277) -> ()  [unwired: 10 in, 1 out]
      }
    }
    n154 = Format Into String(format string="Manager 2.Event Loop\n%s\n", w88) -> (resulting string=w89:string)  [unwired: 2 in, 1 out]
    n155 = call "Error Control.vi"("Command"=ErrorCommand."Set Error", "error in (no error)"=w97, "Source"=w89) -> ()  [unwired: 5 in, 1 out]
    "EventLoop" <- w102
  }
  n156 = call "DisplayQ.vi"("command"=DisplayQCommand."Get Q Reference", "error in (no error)"=w11) -> ("error out"=w13:errorcluster, "queue out"=w14:refnum<queue>)  [unwired: 3 in, 2 out]
  n157 = call "ErrorQ.vi"("command"=DisplayQCommand."Get Q Reference", "error in (no error)"=w11) -> ("error out"=w16:errorcluster, "queue out"=w17:refnum<queue>)  [unwired: 3 in, 2 out]
  n158 = while {
    shift-right: [w289] -> _
    shift-left: w24 -> [w285]
    tunnel: w11 -> [w290]
    tunnel: [-1 ("ErrorHandlingLoop")] -> w22
    tunnel: w3 -> [w280]
    tunnel: w2 -> [w279]
    tunnel: w1 -> [w278]
    i -> [w288]
    stop <- w291 stop-if-true
    (unwired) SetupModeState."Idling"  # State
    (unwired) Transition."No Transition - Error"  # Transition
    # "Use command verbs here"
    # "Use \"-ing\" words here"
    # "4.State Machine (as much as possible in here)"
    n159 = case shown="\"Sorting Menu\"" w285 {
      selector: w285 -> [w311 w338 w397 _ w424 w448 w458 w469]
      tunnel: [_ _ _ _ _ _ _ TRUE] -> w291
      tunnel: w290 -> [w310 w330 w396 w408 w425 w449 w462 w467]
      tunnel: [w320 w339 w390 w413 w415 w439 w461 SetupModeState."No State - Error" ("State 2")] -> w289
      tunnel: [w309 w325 w395 w407 w416 w440 w460 w466] -> w286
      tunnel: w280 -> [w308 w333 _ _ _ _ _ _]
      tunnel: w279 -> [_ w332 _ _ _ _ _ _]
      tunnel: w278 -> [w307 w324 _ w406 _ _ _ w468]
      frame "Initialising", Default {
        w320 = SetupModeState."Idling"  # State
        n160 = call <vilib>:"Application Directory.vi"() -> ("Application Directory"=w295:path)
        n161 = call "DeferPanelUpdates.vi"("error in (no error)"=w310, "Defer Panel Updates"=TRUE, "VI in"=w307) -> ("error out"=w314:errorcluster)  [unwired: 8 in]
        n162 = call "Set State Display.vi"("State"=w311, "error in (no error)"=w314) -> ("error out"=w304:errorcluster)  [unwired: 6 in]
        n163 = Build Path(base path=w295, name or relative path="SourceCode\\SubVIs\\Buttons\\Image") -> (appended path=w293:path)
        n164 = property on="ButtonsMenu" class="TabCtl (strict)"(error in=w304, "Visible"=FALSE) -> (error out=w303:errorcluster)  [unwired: 1 in, 1 out]
        n165 = Build Path(base path=w293, name or relative path="BackgroundTests.vi") -> (appended path=w296:path)
        n166 = Open VI Reference(vi path=w296) -> (vi reference=w299:refnum<vi>, error out=w300:errorcluster)  [unwired: 5 in]
        n167 = call "GetVIPaths.vi"("MenuType"=MenuType."Main", "error in (no error)"=w303) -> ("error out"=w319:errorcluster, "SubMenu VIs"=w317:path[], "Menu VIs"=w316:path[])  [unwired: 4 in]
        n168 = invoke class="VI" method="Run VI"(reference=w299, error in=w300, "Wait until done"=FALSE ("Wait Until Done"), "Auto Dispose Ref"=FALSE ("Auto Dispose Reference")) -> (reference out=w298:refnum<vi>)  [unwired: 1 in, 4 out]
        n169 = control-ref of="Background"() -> (w292:refnum<vi>)
        n170 = call "ButtonControl.vi"("SubPanel Command"=ButtonCommands."Load Buttons", "MenuButtons"=w316, "error in (no error)"=w319, "SubMenuButtons"=w317, "MenuButtonPanels"=w308) -> ("error out"=w312:errorcluster)  [unwired: 5 in]
        n171 = invoke on="Invoke Node" class="SubPnl" method="Insert VI"(reference=w292, "VI Ref"=w298) -> ()  [unwired: 2 in, 4 out]
        n172 = call "DeferPanelUpdates.vi"("error in (no error)"=w312, "Defer Panel Updates"=FALSE, "VI in"=w307) -> ("error out"=w309:errorcluster)  [unwired: 8 in]
      }
      frame "Sorting Menu" {
        w339 = SetupModeState."Idling"  # State
        n173 = call "DeferPanelUpdates.vi"("error in (no error)"=w330, "Defer Panel Updates"=TRUE, "VI in"=w324) -> ("error out"=w329:errorcluster)  [unwired: 8 in]
        n174 = call "Set State Display.vi"("State"=w338, "error in (no error)"=w329) -> ("error out"=w328:errorcluster)  [unwired: 6 in]
        n175 = local read "Menu Output"() -> (w337:string)
        n176 = case shown="\"Developer Tools\"" w337 {
          tunnel: w328 -> [w364 w369 w374 w379 w384 w389]
          tunnel: [w364 w369 w374 w379 w384 w389] -> w322
          tunnel: [MenuType."Main" ("MenuType") MenuType."Main" ("MenuType") MenuType."Simulation" ("MenuType") MenuType."ME" ("MenuType") MenuType."User Utilities" ("MenuType") MenuType."Dev Tools" ("MenuType")] -> w336
          tunnel: [w363 w368 w373 w378 w383 w388] -> w335
          tunnel: [w361 _ _ _ _ _] -> w334
          tunnel: [_ T1 {"Width"=1, "Height"=1} ("Container Bounds") T1 {"Width"=132, "Height"=90} ("Container Bounds") T1 {"Width"=335, "Height"=90} ("Container Bounds") T1 {"Width"=402, "Height"=90} ("Container Bounds") T1 {"Width"=272, "Height"=90} ("Container Bounds")] -> w323
          tunnel: [w360 w365 w370 w375 w380 w385] -> w321
          frame "False", Default {
            w360 = 0  # Position:Top
            w363 = FALSE  # Menu?
            n177 = local read "UI Output"() -> (w361:string)
          }
          frame "Main" {
            w365 = 0  # Position:Top
            w368 = TRUE  # Menu?
          }
          frame "Simulation" {
            w370 = 56  # Position:Top
            w373 = TRUE  # Menu?
          }
          frame "ME" {
            w375 = 130  # Position:Top
            w378 = TRUE  # Menu?
          }
          frame "User Utils" {
            w380 = 320  # Position:Top
            w383 = TRUE  # Menu?
          }
          frame "Developer Tools" {
            w385 = 400  # Position:Top
            w388 = TRUE  # Menu?
          }
        }
        n178 = local write "Container Bounds"(w323) -> ()
        n179 = local write "Position:Top"(w321) -> ()
        n180 = case shown="True" w335 {
          tunnel: [w342 w351] -> w326
          tunnel: w333 -> [_ w353]
          tunnel: w332 -> [_ w357]
          tunnel: w336 -> [_ w354]
          tunnel: w334 -> [w343 _]
          tunnel: w323 -> [_ w349]
          tunnel: w322 -> [w340 w348]
          tunnel: w321 -> [_ w344]
          frame False {
            w341 = FALSE ("Visible")
            # "Not a menu Load a vi"
            n181 = One Button Dialog(message=w343) -> ()  [unwired: 1 in, 1 out]
            n182 = local write "SubmenuVisible"(w341) -> ()
            n183 = property on="ButtonsMenu" class="TabCtl (strict)"(error in=w340, "Visible"=w341) -> (error out=w342:errorcluster)  [unwired: 1 in, 1 out]
          }
          frame True {
            # "Menu"
            n184 = control-ref of="Background"() -> (w350:refnum<vi>)
            n185 = property on="ButtonsMenu" class="TabCtl (strict)"("Top"=w344, "Left"=50 ("Position:Left")) -> ()  [unwired: 2 in, 2 out]
            n186 = property class="SubPnl"(reference=w350, error in=w348, "Container Bounds"=w349) -> (error out=w347:errorcluster)  [unwired: 1 out]
            n187 = local read "SubmenuVisible"() -> (w346:bool)
            n188 = call "GetVIPaths.vi"("MenuType"=w354, "error in (no error)"=w347) -> ("error out"=w359:errorcluster, "SubMenu VIs"=w356:path[], "Menu VIs"=w355:path[])  [unwired: 4 in]
            n189 = call "ButtonControl.vi"("SubPanel Command"=ButtonCommands."Load Buttons", "MenuButtons"=w355, "error in (no error)"=w359, "SubMenuButtons"=w356, "SubMenuButtonPanels"=w357, "MenuButtonPanels"=w353) -> ("error out"=w352:errorcluster)  [unwired: 4 in]
            n190 = property on="ButtonsMenu" class="TabCtl (strict)"(error in=w352, "Visible"=w346) -> (error out=w351:errorcluster)  [unwired: 1 in, 1 out]
          }
        }
        n191 = call "DeferPanelUpdates.vi"("error in (no error)"=w326, "Defer Panel Updates"=FALSE, "VI in"=w324) -> ("error out"=w325:errorcluster)  [unwired: 8 in]
      }
      frame "Sorting Submenu" {
        n192 = call "Set State Display.vi"("State"=w397, "error in (no error)"=w396) -> ("error out"=w393:errorcluster)  [unwired: 6 in]
        n193 = local read "UI Output"() -> (w391:string)
        n194 = case shown="\"Close Screen\"" w391 {
          tunnel: w393 -> [w399 w402]
          tunnel: [w399 w401] -> w392
          tunnel: [w398 SetupModeState."Exiting" ("State")] -> w390
          frame "False", Default {
            w398 = SetupModeState."Idling"  # State
          }
          frame "Close Screen" {
            n195 = property on="exit" class="Bool (strict)"(error in=w402, "Val(Sgnl)"=TRUE ("Value (Signaling)")) -> (error out=w401:errorcluster)  [unwired: 1 in, 1 out]
          }
        }
        n196 = local read "SubmenuVisible"() -> (w394:bool)
        n197 = property on="ButtonsMenu" class="TabCtl (strict)"(error in=w392, "Visible"=w394) -> (error out=w395:errorcluster)  [unwired: 1 in, 1 out]
      }
      frame "Resetting Menu" {
        w413 = SetupModeState."Sorting Menu"  # State
        n198 = call "DeferPanelUpdates.vi"("error in (no error)"=w408, "Defer Panel Updates"=TRUE, "VI in"=w406) -> ("error out"=w404:errorcluster)  [unwired: 8 in]
        n199 = call "ButtonControl.vi"("SubPanel Command"=ButtonCommands."Remove Buttons", "error in (no error)"=w404) -> ("error out"=w409:errorcluster)  [unwired: 8 in]
        n200 = call <vilib>:"Clear Errors.vi"("error in (no error)"=w409) -> ("error out"=w405:errorcluster)  [unwired: 5 in, 1 out]
        n201 = call "DeferPanelUpdates.vi"("error in (no error)"=w405, "Defer Panel Updates"=FALSE, "VI in"=w406) -> ("error out"=w407:errorcluster)  [unwired: 8 in]
      }
      frame "Idling" {
        # "Transition"
        # "State"
        n202 = call "Set State Display.vi"("State"=w424, "error in (no error)"=w425) -> ("error out"=w419:errorcluster)  [unwired: 6 in]
        n203 = call "StateQ.vi"("QueueCommand"=QueueCommand."Get Ref", "error in (no error)"=w419) -> ("error out"=w421:errorcluster, "queue out"=w420:refnum<queue>)  [unwired: 5 in]
        n204 = Dequeue Element(queue=w420, error in (no error)=w421) -> (element=w423:T11, error out=w418:errorcluster)  [unwired: 1 in, 2 out]
        n205 = Unbundle By Name(w423) -> ("Transition"=w417:T12, "variant"=w414:variant)
        n206 = case shown="\"Menu Button Pressed\"" w417 {
          tunnel: [SetupModeState."Idling" ("State 2") SetupModeState."Running" ("State 2") SetupModeState."Sorting Submenu" ("State 2") SetupModeState."Resetting Menu" ("State 2") SetupModeState."Erroring" ("State 2") SetupModeState."Exiting" ("State 2")] -> w415
          tunnel: w418 -> [w426 w428 w430 w432 _ w436]
          tunnel: [w426 w428 w430 w432 errorcluster {"status"=TRUE, "code"=99998, "source"="State Error"} ("error out") w436] -> w416
          tunnel: w414 -> [_ _ _ _ _ _]
          frame "No Transition - Error", Default {
            # "Can Trap This"
          }
          frame "Start" {
          }
          frame "UI Button Pressed" {
          }
          frame "Menu Button Pressed" {
          }
          frame "Generate Error" {
          }
          frame "Exit" {
          }
        }
      }
      frame "Running" {
        # "Transition"
        # "State"
        n207 = call "Set State Display.vi"("State"=w448, "error in (no error)"=w449) -> ("error out"=w443:errorcluster)  [unwired: 6 in]
        n208 = call "StateQ.vi"("QueueCommand"=QueueCommand."Get Ref", "error in (no error)"=w443) -> ("error out"=w445:errorcluster, "queue out"=w444:refnum<queue>)  [unwired: 5 in]
        n209 = Dequeue Element(queue=w444, error in (no error)=w445) -> (element=w447:T11, error out=w442:errorcluster)  [unwired: 1 in, 2 out]
        n210 = Unbundle By Name(w447) -> ("Transition"=w441:T12, "variant"=w438:variant)
        n211 = case shown="\"Stop\"" w441 {
          tunnel: [SetupModeState."Idling" ("State 2") SetupModeState."Idling" ("State 2") SetupModeState."Erroring" ("State 2") SetupModeState."Exiting" ("State 2")] -> w439
          tunnel: w442 -> [w450 w452 _ w456]
          tunnel: [w450 w452 errorcluster {"status"=TRUE, "code"=99998, "source"="State Error"} ("error out") w456] -> w440
          tunnel: w438 -> [_ _ _ _]
          frame "No Transition - Error", Default {
            # "Can Trap This"
          }
          frame "Stop" {
          }
          frame "Generate Error" {
          }
          frame "Exit" {
          }
        }
      }
      frame "Erroring" {
        # "Transition"
        # "State"
        n212 = call "Set State Display.vi"("State"=w458, "error in (no error)"=w462) -> ("error out"=w459:errorcluster)  [unwired: 6 in]
        n213 = call "WaitForTransition.vi"("error in (no error)"=w459, "State"=w458) -> ("error out"=w460:errorcluster, "StateOut"=w461:T2)  [unwired: 4 in]
      }
      frame "Exiting" {
        n214 = call "DeferPanelUpdates.vi"("error in (no error)"=w467, "Defer Panel Updates"=TRUE, "VI in"=w468) -> ("error out"=w472:errorcluster)  [unwired: 8 in]
        n215 = call "Set State Display.vi"("State"=w469, "error in (no error)"=w472) -> ("error out"=w464:errorcluster)  [unwired: 6 in]
        n216 = property on="ButtonsMenu" class="TabCtl (strict)"(error in=w464, "Visible"=FALSE) -> (error out=w463:errorcluster)  [unwired: 1 in, 1 out]
        n217 = call "ButtonControl.vi"("SubPanel Command"=ButtonCommands."Remove Buttons", "error in (no error)"=w463) -> ("error out"=w470:errorcluster)  [unwired: 8 in]
        n218 = call "DeferPanelUpdates.vi"("error in (no error)"=w470, "Defer Panel Updates"=FALSE, "VI in"=w468) -> ("error out"=w466:errorcluster)  [unwired: 8 in]
      }
    }
    n219 = Format Into String(format string="%s", initial string="4.State Machine\n", w285) -> (resulting string=w284:string)  [unwired: 1 in, 1 out]
    n220 = call "Error Control.vi"("Command"=ErrorCommand."Set Error", "error in (no error)"=w286, "Source"=w284) -> ()  [unwired: 5 in, 1 out]
    "StateMachineLoop" <- w288
    "State" <- w285
  }
  n221 = while {
    tunnel: w16 -> [w487]
    tunnel: w17 -> [w486]
    tunnel: [w478] -> w4
    tunnel: [-1 ("ErrorHandlingLoop")] -> w23
    i -> [w480]
    stop <- w481 stop-if-true
    (unwired) DisplayMessage."No Message - Ignore" ("DisplayMessage")
    # "5. Error Handling"
    n222 = Dequeue Element(queue=w486, error in (no error)=w487) -> (element=w485:cluster{"ErrorMessage":T10, "DataIn":variant}, error out=w482:errorcluster)  [unwired: 1 in, 2 out]
    n223 = Unbundle By Name(w485) -> ("ErrorMessage"=w483:T10, "DataIn"=w484:variant)
    n224 = case shown="\"Display Message\"" w483 {
      tunnel: w484 -> [_ w504 _]
      tunnel: w482 -> [w488 w503 w507]
      tunnel: [w488 w494 w507] -> w478
      tunnel: [_ FALSE ("STOP?") TRUE ("STOP?")] -> w481
      tunnel: string[] [] -> [_ w502 _]
      frame "No Message - Ignore", Default {
        n225 = Wait (ms)(milliseconds to wait=u32 1) -> ()  [unwired: 1 out]
      }
      frame "Display Message" {
        n226 = Variant To Data(error in=w503, type=w502, Variant=w504) -> (data=w496:string[], error out=w495:errorcluster)
        n227 = Get Date/Time String(date format (0)=enum16{"short", "long", "abbreviated"}."short", want seconds? (F)=TRUE) -> (date string=w499:string, time string=w498:string)  [unwired: 1 in]
        n228 = Concatenate Strings(w499, " " ("string"), w498) -> (w490:string)
        "Error" <- w490
        n229 = Build Array (concatenate)(w490, w496) -> (w491:string[])
        n230 = call "DisplayQ.vi"("command"=DisplayQCommand."Add Item to Bottom", "error in (no error)"=w495, "DataIn"=w491, "DisplayMessage"=DisplayMessage."Add Error Message") -> ("error out"=w494:errorcluster)  [unwired: 1 in, 3 out]
      }
      frame "Stop" {
      }
    }
    "ErrorHandlingLoop" <- w480
  }
  n231 = while "3. User Interface Queue Handling" {
    tunnel: w13 -> [w522]
    tunnel: w14 -> [w521]
    tunnel: [-1 ("ErrorHandlingLoop")] -> w21
    i -> [w513]
    stop <- w514 stop-if-true
    (unwired) DisplayMessage."No Message - Ignore" ("DisplayMessage")
    # "Add New UI Stuff Here"
    # "3. User Interface Queue Handling (Only update controls and indicators in here)"
    n232 = Dequeue Element(queue=w521, error in (no error)=w522) -> (element=w520:cluster{"DisplayMessage":T9, "DataIn":variant}, error out=w517:errorcluster)  [unwired: 1 in, 2 out]
    n233 = Unbundle By Name(w520) -> ("DisplayMessage"=w518:T9, "DataIn"=w519:variant)
    n234 = case shown="\"Set Subpanel Output\"" w518 {
      selector: w518 -> [w523 w526 w529 w544 w551 w555 w559 w561 w563 w583]
      tunnel: w519 -> [_ _ w538 w547 _ _ _ _ w567 w569]
      tunnel: w517 -> [w524 w528 w531 w546 w550 w554 w558 _ w565 w570]
      tunnel: [w524 w528 w530 w545 w550 w554 w558 errorcluster {"status"=TRUE, "code"=99997, "source"="UI Error"} ("error out") w564 w568] -> w516
      tunnel: [_ TRUE ("STOP?") _ _ _ _ _ _ _ _] -> w514
      tunnel: [w523 w526 w529 w544 w551 w555 w559 w561 w563 w583] -> w512
      frame "No Message - Ignore", Default {
        n235 = Wait (ms)(milliseconds to wait=u32 1) -> ()  [unwired: 1 out]
      }
      frame "Stop" {
      }
      frame "Display Message" {
        n236 = Variant To Data(error in=w531, type="" ("data"), Variant=w538) -> (data=w534:string, error out=w530:errorcluster)
        n237 = local read "State"() -> (w536:T2)
        n238 = Format Into String(w536) -> (resulting string=w535:string)  [unwired: 3 in, 1 out]
        n239 = Concatenate Strings(w535, " - " ("string"), w534) -> (→"Status":string)
      }
      frame "Add Error Message" {
        n240 = property on="ErrorLog" class="MCListbox (strict)"() -> ("ItemNames"=w542:string[][])  [unwired: 2 in, 2 out]
        n241 = Variant To Data(error in=w546, type=string[] [], Variant=w547) -> (data=w541:string[], error out=w545:errorcluster)
        n242 = Build Array (concatenate)(w542, w541) -> (w539:string[][])
        n243 = property on="ErrorLog" class="MCListbox (strict)"("ItemNames"=w539) -> ()  [unwired: 2 in, 2 out]
        "ErrorIndicator" <- TRUE ("ErrorIndicator")
      }
      frame "Set Idling Display" {
        w548 = FALSE  # Visible
        w549 = TRUE  # Visible
        n244 = property on="Stop" class="Bool (strict)"("Visible"=w548) -> ()  [unwired: 2 in, 2 out]
        n245 = property on="Start" class="Bool (strict)"("Visible"=w549) -> ()  [unwired: 2 in, 2 out]
      }
      frame "Set Running Display" {
        w552 = TRUE  # Visible
        w553 = FALSE  # Visible
        n246 = property on="Stop" class="Bool (strict)"("Visible"=w552) -> ()  [unwired: 2 in, 2 out]
        n247 = property on="Start" class="Bool (strict)"("Visible"=w553) -> ()  [unwired: 2 in, 2 out]
      }
      frame "Clear Error History" {
        n248 = property on="ErrorLog" class="MCListbox (strict)"("ItemNames"=string[][] []) -> ()  [unwired: 2 in, 2 out]
        n249 = local write "ErrorIndicator"(FALSE ("ErrorIndicator")) -> ()
      }
      frame "Generate Error" {
      }
      frame "Set Tab" {
        n250 = Variant To Data(error in=w565, type=Tab."Eng Run Screen" ("Tab Control"), Variant=w567) -> (data=→"Tab Control":T15, error out=w564:errorcluster)
      }
      frame "Set Subpanel Output" {
        n251 = Variant To Data(error in=w570, type="", Variant=w569) -> (data=w582:string, error out=w575:errorcluster)
        n252 = Match Pattern(string=w582, regular expression=":") -> (after substring=w581:string, offset past match=w577:i32)  [unwired: 1 in, 2 out]
        n253 = Less Than 0?(x=w577) -> (x < 0?=w578:bool)
        n254 = case shown="True" w578 {
          tunnel: w581 -> [w587 _]
          tunnel: [Transition."Menu Button Pressed" ("Transition") Transition."UI Button Pressed" ("Transition")] -> w579
          tunnel: [w586 w591] -> w580
          tunnel: w582 -> [_ w591]
          frame False {
            # "Menu"
            n255 = local read "Menu Output"() -> (w589:string)
            n256 = Equal?(x=w589, y=w587) -> (x = y?=w585:bool)
            n257 = Not(x=w585) -> (.not. x?=→"SubmenuVisible":bool)
            n258 = Select(t="Main", s=w585, f=w587) -> (s? t:f=w586:string)
            "Menu Output" <- w586
          }
          frame True {
            # "UI"
            "UI Output" <- w591
          }
        }
        n259 = Bundle By Name(cluster=T11 {"Transition"=enum."No Transition - Error", "variant"=variant} ("output cluster"), "Transition"=w579, "variant"=w580) -> (w576:T11)
        n260 = call "StateQ.vi"("QueueCommand"=QueueCommand."Add to Bottom", "error in (no error)"=w575, "output cluster"=w576) -> ("error out"=w568:errorcluster)  [unwired: 4 in, 1 out]
      }
    }
    n261 = Format Into String(format string="%s", initial string="3.UI Queue Handling\n", w512) -> (resulting string=w511:string)  [unwired: 1 in, 1 out]
    n262 = call "Error Control.vi"("Command"=ErrorCommand."Set Error", "error in (no error)"=w516, "Source"=w511) -> ()  [unwired: 5 in, 1 out]
    "UILoop" <- w513
  }
  n263 = local write "ErrorHandlingLoop"(w23) -> ()
  n264 = call "DisplayQ.vi"("command"=DisplayQCommand."Close", "error in (no error)"=w4) -> ("error out"=w6:errorcluster)  [unwired: 3 in, 3 out]
  n265 = call "StateQ.vi"("QueueCommand"=QueueCommand."Close", "error in (no error)"=w6) -> ("error out"=w8:errorcluster)  [unwired: 5 in, 1 out]
  n266 = local write "EventLoop"(w20) -> ()
  n267 = call "ErrorQ.vi"("command"=DisplayQCommand."Close", "error in (no error)"=w8) -> ("error out"=w9:errorcluster)  [unwired: 3 in, 3 out]
  n268 = call "SSDCExit.vi"("error in (no error)"=w9) -> ()  [unwired: 6 in, 1 out]
  n269 = local write "StateMachineLoop"(w22) -> ()
  n270 = local write "UILoop"(w21) -> ()
